vi "Write.vi"(8 "error in (no error)":errorcluster, 9 "timeout ms (25000)":i32, 10 "Bytes to write":u8[](array[numeric]), 11 "VISA TCP in":refnum<class "VISA TCP.lvclass">) -> (0 "error out":errorcluster, 2 "bytes written":i32, 3 "VISA TCP out":refnum<class "VISA TCP.lvclass">)   [LabVIEW 2013, in "Sockets.lvlib" / "VISA TCP.lvclass"]
doc: "Writes data to the socket."
uses:
  VISA TCP.lvclass
  VISA TCP.lvclass/VISA TCP.ctl
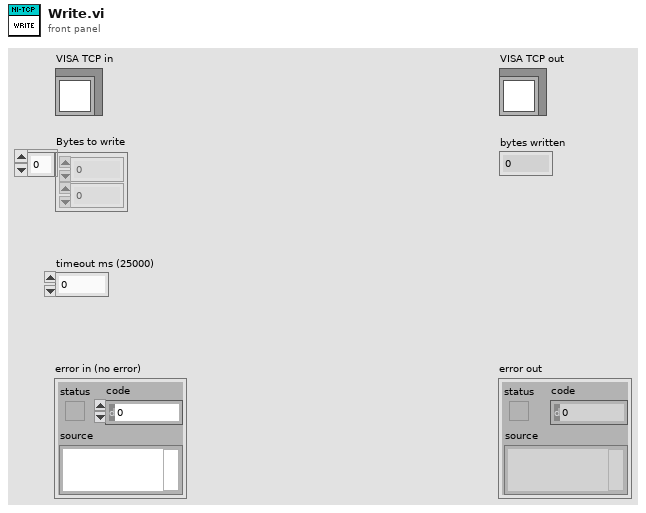
[diagram p1: front panel]
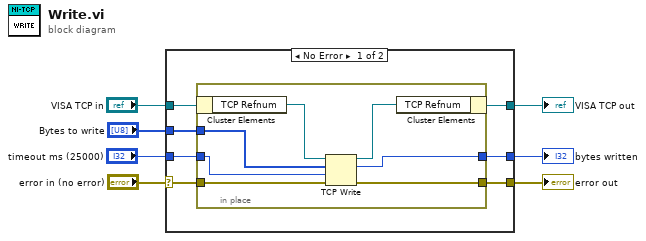
[diagram p0: block diagram]
diagram:
  n1 = case shown="No Error" "error in (no error)" {
    selector: "error in (no error)" -> [w9 w23]
    tunnel: "VISA TCP in" -> [w14 w22]
    tunnel: [w13 w22] -> w4
    tunnel: [w12 w23] -> w6
    tunnel: "timeout ms (25000)" -> [w11 _]
    tunnel: "Bytes to write" -> [w10 _]
    tunnel: [w8 _] -> w3
    frame No Error {
      n2 = in-place {
        in-place-border: w9 -> [w19]
        in-place-border: [w18] -> w12
        in-place-border: w10 -> [w17]
        in-place-border: w11 -> [w16]
        in-place-border: [w15] -> w8
        n3 = in-place-cluster #1(w14) -> ("TCP Refnum"=w21:refnum<k5>)
        n4 = TCP Write(connection ID=w21, data in=w17, error in (no error)=w19, 9:w16) -> (connection ID out=w20:refnum<k5>, bytes written=w15:i32, error out=w18:errorcluster)
        n5 = in-place-cluster #1("TCP Refnum"=w20) -> (w13:refnum<class "VISA TCP.lvclass">)
      }
    }
    frame Error {
    }
  }
  "error out" <- w6
  "VISA TCP out" <- w4
  "bytes written" <- w3
